vi "SetStreamInfo.vi"(8 "error in (no error)":errorcluster, 9 "block":i32, 10 "SendEventRef":T1, 11 "data in":variant) -> (0 "error out":errorcluster, 3 "data out":variant)   [LabVIEW 2017, in "FileManager.lvlib"]
uses:
  <vilib>/addons/InsightCM/Devices/Shared/Common/FileManager/FileManager.lvlib
  <vilib>/addons/InsightCM/Devices/Shared/Common/FileManager/controls/SendEventRefRoutedMessage.ctl
  <vilib>/addons/InsightCM/Devices/Shared/Common/DataEvent/controls/EventReference.ctl
  <vilib>/addons/InsightCM/Devices/Shared/Common/DataEvent/controls/Event.ctl
  <vilib>/addons/InsightCM/MessageBus/Base/controls/DataEvent.ctl
  <vilib>/addons/InsightCM/MessageBus/Base/controls/KeyValuePair.ctl
  <vilib>/addons/InsightCM/Devices/Shared/Common/DataEvent/controls/DataSet.ctl
  <vilib>/addons/InsightCM/MessageBus/Base/controls/DataSetMetadata.ctl
  <vilib>/addons/InsightCM/MessageBus/Base/controls/TrendPoint.ctl
  <vilib>/addons/InsightCM/MessageBus/Base/controls/TrendAlarmUpdate.ctl
  <vilib>/addons/InsightCM/MessageBus/Base/controls/TrendAlarmTransition.ctl
  <vilib>/addons/InsightCM/Devices/Shared/Common/DataEvent/DataEvent.lvlib
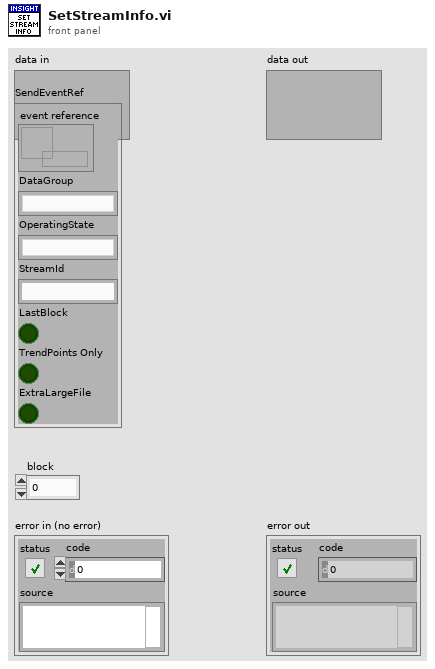
[diagram p1: front panel]
types:
  T1 = typedef "FileManager.lvlib/SendEventRefRoutedMessage.ctl" = cluster{"event reference":T2, "DataGroup":string, "OperatingState":string, "StreamId":string, "LastBlock":bool, "TrendPoints Only":bool, "ExtraLargeFile":bool}
  T2 = typedef "DataEvent.lvlib/EventReference.ctl" = refnum<data-value>
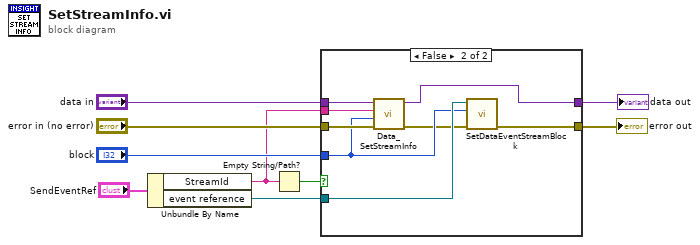
[diagram p0: block diagram]
diagram:
  n1 = Unbundle By Name("SendEventRef") -> ("StreamId"=w1:string, "event reference"=w3:T2)
  n2 = Empty String/Path?(string/path=w1) -> (empty?=w2:bool)
  n3 = case shown="False" w2 {
    tunnel: "error in (no error)" -> [w10 w16]
    tunnel: "data in" -> [w11 w18]
    tunnel: [w10 w12] -> w7
    tunnel: [w11 w17] -> w6
    tunnel: "block" -> [_ w14]
    tunnel: w3 -> [_ w19]
    tunnel: w1 -> [_ w15]
    frame True {
      # "If StreamId is empty, this is not a stream"
    }
    frame False {
      n4 = call <vilib>:"Data_SetStreamInfo.vi"("error in (no error)"=w16, "block"=w14, "streamId"=w15, "data in"=w18) -> ("error out"=w13:errorcluster, "data out"=w17:variant)  [unwired: 6 in]
      n5 = call <vilib>:"SetDataEventStreamBlock.vi"("error in (no error)"=w13, "block"=w14, "data event reference"=w19) -> ("error out"=w12:errorcluster)  [unwired: 8 in]
    }
  }
  "error out" <- w7
  "data out" <- w6
